vi "Temp1.vi"() -> ()   [LabVIEW 2018]
uses:
  <vilib>/Instr/_visa.llb/VISA Configure Serial Port (Instr).vi
panel:
  in  "String":string
  out "error out":errorcluster
  in  "error in (no error)":errorcluster
  out "String 2":string
  in  "VISA resource name":refnum<visa-resource-name>
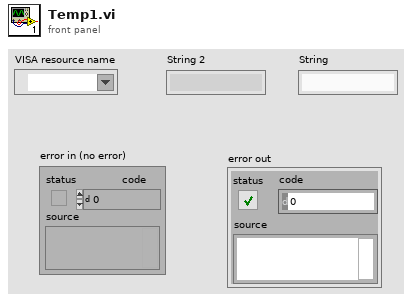
[diagram p1: front panel]
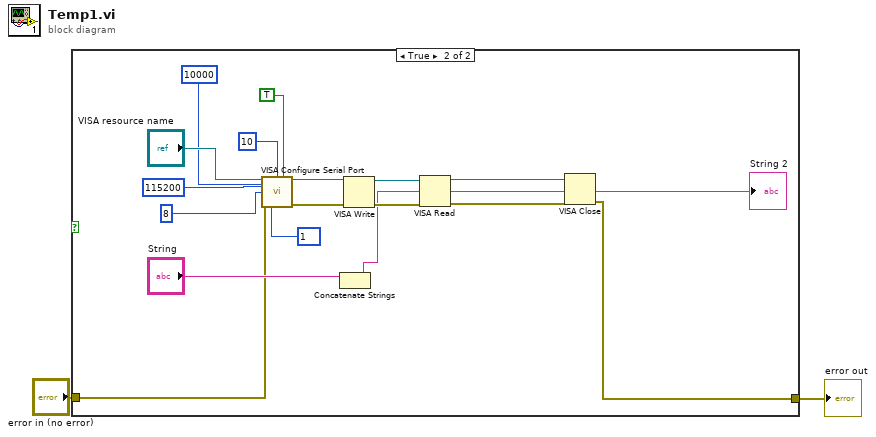
[diagram p0: block diagram]
diagram:
  n1 = case shown="True" {
    selector: _ -> [_ _]
    tunnel: "error in (no error)" -> [_ w7]
    tunnel: [_ w6] -> w1
    frame False {
    }
    frame True {
      w16 = u16 10 items=["1"=10, "1.5"=15, "2.0"=20] ("stop bits (10: 1 bit)")
      n2 = call-poly "VISA Configure Serial Port"("VISA resource name"="VISA resource name", "timeout (10sec)"=u32 10000, "termination char\n(0xA = '\\n' = LF)"=u8 10 ("termination char\n(0xA = '\\n' = LF)"), "Enable Termination\nChar (T)"=TRUE ("Enable Termination\nChar (T)"), "baud rate (9600)"=115200, "data bits (8)"=8, "error in (no error)"=w7, "stop bits (10: 1 bit)"=w16) -> ("VISA resource name out"=w15:refnum<visa-resource-name>, "error out"=w12:errorcluster)  [unwired: 6 in]
      n3 = Concatenate Strings("String") -> (→"String 2":string)  [unwired: 1 in]
      n4 = VISA Write(VISA resource name=w15, error in (no error)=w12) -> (VISA resource name out=w14:refnum<visa-resource-name>, error out=w11:errorcluster)  [unwired: 1 in, 1 out]
      n5 = VISA Read(VISA resource name=w14, error in (no error)=w11) -> (VISA resource name out=w13:refnum<visa-resource-name>, error out=w10:errorcluster)  [unwired: 1 in, 2 out]
      n6 = VISA Close(VISA resource name=w13, error in (no error)=w10) -> (error out=w6:errorcluster)
    }
  }
  "error out" <- w1
